vi "ZCAN_StartLIN.vi"(8 "error in (no error)":errorcluster caption="错误输入（无错误）", 10 "lin_index_handle":u32) -> (0 "error out":errorcluster caption="错误输出", 1 "lin_index_handle(out)":u32, 2 "startcan_success?":bool)   [LabVIEW 2020, in "zlgcan.lvlib"]
uses:
  zlgcan.lvlib
  bin/zlgcan_wrap.dll
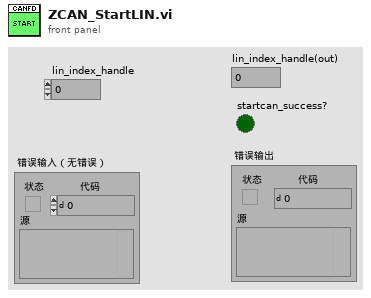
[diagram p1: front panel]
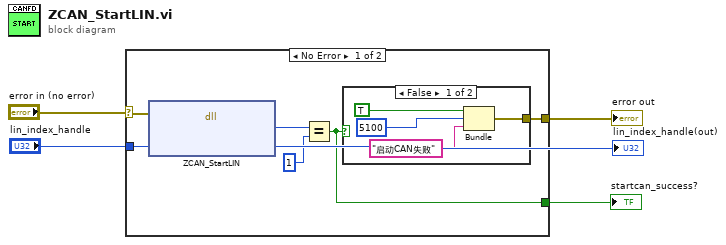
[diagram p0: block diagram]
diagram:
  n1 = case shown="No Error" "error in (no error)" {
    selector: "error in (no error)" -> [w8 w15]
    tunnel: [w6 w15] -> w3
    tunnel: "lin_index_handle" -> [w7 _]
    tunnel: [w5 _] -> w2
    frame No Error {
      n2 = dll-call lib="E:/Jabil tools/JabilTestLib/ZLG_CANFD/bin/zlgcan_wrap.dll" fn="ZCAN_StartLIN" ("ZCAN_StartCAN")(error in=w8, "can_handle"=w7) -> ("return"=w10:u32)  [unwired: 3 in, 2 out]
      n3 = Equal?(x=w10, y=1) -> (x = y?=w5:bool)
      n4 = case shown="False" w5 {
        tunnel: [w11 _] -> w6
        frame False {
          n5 = Bundle("status"=TRUE, "code"=5100, "消息"="启动CAN失败") -> (w11:cluster{"status":bool, "code":i32, "消息":string})  [unwired: 1 in]
        }
        frame True {
        }
      }
    }
    frame Error {
    }
  }
  "error out" <- w3
  "startcan_success?" <- w2
  "lin_index_handle(out)" <- "lin_index_handle"
